vi "REC_ThermalCAM.vi"() -> ()   [LabVIEW 2018]
doc: "To use this browser, you can type in a URL in the location field and then click on the Go button. You can also use the Back, Forward, Reload and Search buttons. This VI also has a runtime menu which is included in the library. When you run the VI, you will have File Menu and a History Menu. The file menu contains the same functionality that the buttons can do and the History menu contains a History of all the pages that you have visited in a given session.\n\nThe Invoke Node and Property Node functions are used to control the operation of the web browser. For more information on the Microsoft Web Browser Control, see Microsoft's web site (try http://support.microsoft.com/support/kb/articles/q165/2/12.asp)."
panel:
  out "Passing Array":string[](array[string])=["http://espn.go.com/", "http://www.natinst.com/"]
  in  "Search":bool
  in  "Go":bool
  in  "Reload":bool
  in  "Back":bool
  in  "Forward":bool
  in  "URL :":string="192.168.1.65"
  in  "SHDocVw.IWebBrowser2":refnum<k7>(container)
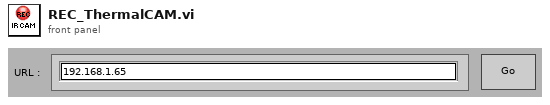
[diagram p1: front panel]
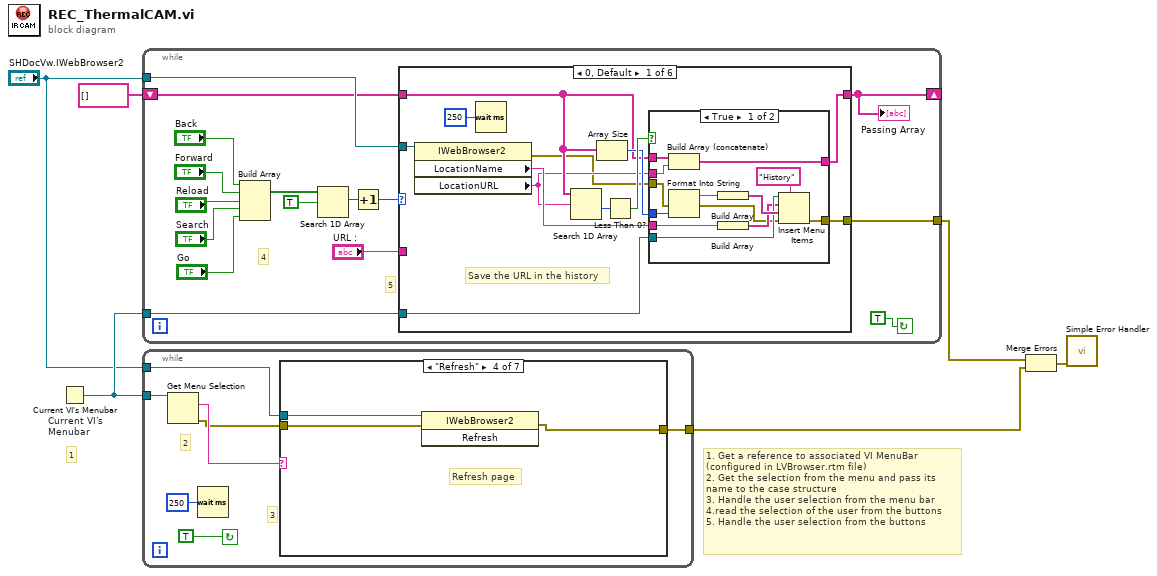
[diagram p0: block diagram]
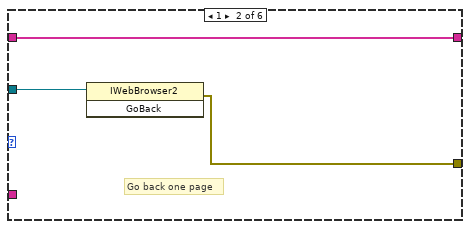
[diagram p3: hidden frame]
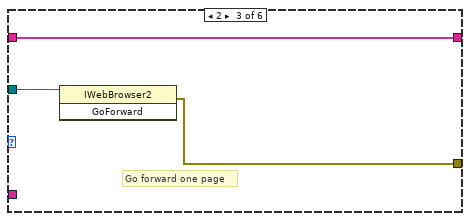
[diagram p4: hidden frame]
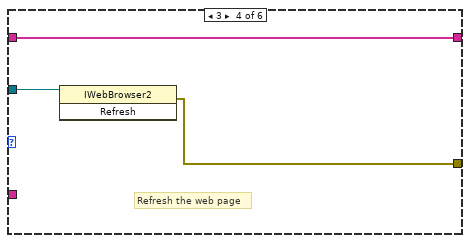
[diagram p5: hidden frame]
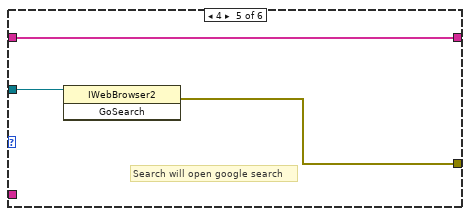
[diagram p6: hidden frame]
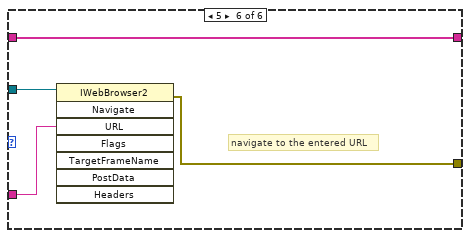
[diagram p7: hidden frame]
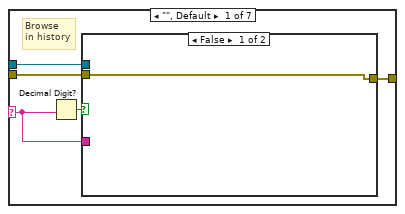
[diagram p8: hidden frame]
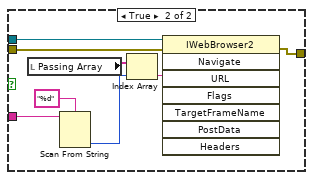
[diagram p9: hidden frame]
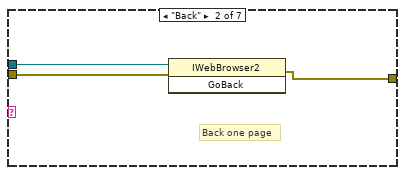
[diagram p10: hidden frame]
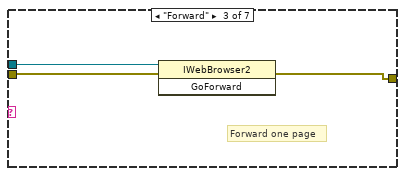
[diagram p11: hidden frame]
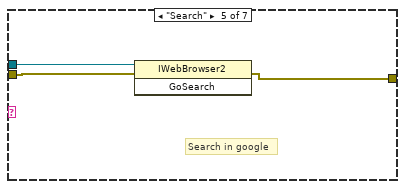
[diagram p12: hidden frame]
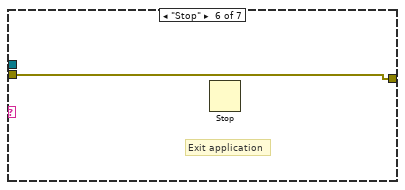
[diagram p13: hidden frame]
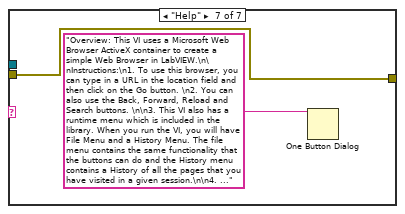
[diagram p14: hidden frame]
diagram:
  # "1. Get a reference to associated VI MenuBar \n(configured in LVBrowser.rtm file)\n2. Get the selection from the menu and pass its \nname to the case structure\n3. Handle the user selection from the menu bar\n4.read the selection of the user from the buttons\n5. Handle the user selection from the buttons"
  # "1"
  n1 = Current VI's Menubar "Current VI's \nMenubar"() -> (w6:refnum<k9>)
  n2 = while {
    shift-left: string[] [] -> [w9]
    shift-right: [w8] -> _
    tunnel: w6 -> [w10]
    tunnel: "SHDocVw.IWebBrowser2" -> [w12]
    tunnel: [w7] -> w3
    stop <- TRUE continue-if-true
    # "5"
    # "4"
    n3 = Build Array("Back", "Forward", "Reload", "Search", "Go") -> (w16:bool[])
    n4 = Search 1D Array(1D array=w16, element=TRUE) -> (index of element=w14:i32)  [unwired: 1 in]
    n5 = Increment(x=w14) -> (x+1=w13:i32)
    n6 = case shown="0, Default" w13 {
      tunnel: w12 -> [w25 w52 w55 w57 w60 w65]
      tunnel: "URL :" -> [_ _ _ _ _ w64]
      tunnel: w10 -> [w26 _ _ _ _ _]
      tunnel: w9 -> [w30 w51 w54 w58 w61 w63]
      tunnel: [w29 w51 w54 w58 w61 w63] -> w8
      tunnel: [w24 w50 w53 w56 w59 w62] -> w7
      frame 0, Default {
        # "Save the URL in the history"
        n7 = property class="IWebBrowser2"(reference=w25) -> (error out=w23:errorcluster, "LocationName"=w34:string, "LocationURL"=w27:string)  [unwired: 1 in, 1 out]
        n8 = Wait (ms)(milliseconds to wait=u32 250 ("millisecond multiple")) -> ()  [unwired: 1 out]
        n9 = Search 1D Array(1D array=w30, element=w27) -> (index of element=w33:i32)  [unwired: 1 in]
        n10 = Array Size(array=w30) -> (size(s)=w31:i32)
        n11 = Less Than 0?(x=w33) -> (x < 0?=w32:bool)
        n12 = case shown="True" w32 {
          tunnel: w26 -> [w44 _]
          tunnel: w34 -> [w42 _]
          tunnel: w27 -> [w38 _]
          tunnel: w31 -> [w39 _]
          tunnel: w30 -> [w41 w49]
          tunnel: [w40 w49] -> w29
          tunnel: [w36 w48] -> w24
          tunnel: w23 -> [w35 w48]
          frame True {
            n13 = Build Array (concatenate)(w41, w38) -> (w40:string[])
            n14 = Format Into String(error in=w35, w39) -> (resulting string=w47:string, error out=w37:errorcluster)  [unwired: 2 in]
            n15 = Build Array(w47) -> (w46:string[])
            n16 = Build Array(w42) -> (w43:string[])
            n17 = Insert Menu Items(5:"History" ("menu tag"), 6:w37, 7:w46, 8:w43, 9:w44) -> (0:w36:errorcluster)  [unwired: 1 in, 2 out]
          }
          frame False {
          }
        }
      }
      frame 1 {
        # "Go back one page"
        n18 = invoke class="IWebBrowser2" method="GoBack"(reference=w52) -> (error out=w50:errorcluster)  [unwired: 2 in, 2 out]
      }
      frame 2 {
        # "Go forward one page"
        n19 = invoke class="IWebBrowser2" method="GoForward"(reference=w55) -> (error out=w53:errorcluster)  [unwired: 2 in, 2 out]
      }
      frame 3 {
        # "Refresh the web page"
        n20 = invoke class="IWebBrowser2" method="Refresh"(reference=w57) -> (error out=w56:errorcluster)  [unwired: 2 in, 2 out]
      }
      frame 4 {
        # "Search will open google search"
        n21 = invoke class="IWebBrowser2" method="GoSearch"(reference=w60) -> (error out=w59:errorcluster)  [unwired: 2 in, 2 out]
      }
      frame 5 {
        # "navigate to the entered URL"
        n22 = invoke class="IWebBrowser2" method="Navigate"(reference=w65, "URL"=w64) -> (error out=w62:errorcluster)  [unwired: 6 in, 7 out]
      }
    }
    "Passing Array" <- w8
  }
  n23 = while {
    tunnel: w6 -> [w71]
    tunnel: "SHDocVw.IWebBrowser2" -> [w69]
    tunnel: [w66] -> w2
    stop <- TRUE continue-if-true
    # "3"
    # "2"
    n24 = Get Menu Selection(0:w71) -> (6:w70:string, 8:w67:errorcluster)  [unwired: 3 in, 3 out]
    n25 = Wait (ms)(milliseconds to wait=u32 250 ("millisecond multiple")) -> ()  [unwired: 1 out]
    n26 = case shown="\"Refresh\"" w70 {
      selector: w70 -> [w75 _ _ _ _ _ _]
      tunnel: w69 -> [w77 w89 w92 w95 w98 _ _]
      tunnel: w67 -> [w74 w88 w91 w94 w97 w99 w100]
      tunnel: [w73 w87 w90 w93 w96 w99 w100] -> w66
      frame "", Default {
        # "Browse\nin history"
        n27 = Decimal Digit?(1:w75) -> (0:w76:bool)
        n28 = case shown="False" w76 {
          tunnel: w77 -> [_ w86]
          tunnel: w75 -> [_ w82]
          tunnel: w74 -> [w78 w80]
          tunnel: [w78 w79] -> w73
          frame False {
          }
          frame True {
            n29 = local read "Passing Array"() -> (w85:string[])
            n30 = Scan From String(format string="%d", input string=w82) -> (output 1=w81:i32)  [unwired: 3 in, 3 out]
            n31 = Index Array(array=w85, index=w81) -> (element=w84:string)
            n32 = invoke class="IWebBrowser2" method="Navigate"(reference=w86, error in=w80, "URL"=w84) -> (error out=w79:errorcluster)  [unwired: 5 in, 7 out]
          }
        }
      }
      frame "Back" {
        # "Back one page"
        n33 = invoke class="IWebBrowser2" method="GoBack"(reference=w89, error in=w88) -> (error out=w87:errorcluster)  [unwired: 1 in, 2 out]
      }
      frame "Forward" {
        # "Forward one page"
        n34 = invoke class="IWebBrowser2" method="GoForward"(reference=w92, error in=w91) -> (error out=w90:errorcluster)  [unwired: 1 in, 2 out]
      }
      frame "Refresh" {
        # "Refresh page"
        n35 = invoke class="IWebBrowser2" method="Refresh"(reference=w95, error in=w94) -> (error out=w93:errorcluster)  [unwired: 1 in, 2 out]
      }
      frame "Search" {
        # "Search in google"
        n36 = invoke class="IWebBrowser2" method="GoSearch"(reference=w98, error in=w97) -> (error out=w96:errorcluster)  [unwired: 1 in, 2 out]
      }
      frame "Stop" {
        # "Exit application"
        n37 = Stop() -> ()  [unwired: 1 in]
      }
      frame "Help" {
        n38 = One Button Dialog(message="Overview: This VI uses a Microsoft Web Browser ActiveX container to create a simple Web Browser in LabVIEW.\n\nInstructions:\n1. To use this browser, you can type in a URL in the location field and then click on the Go button. \n2. You can also use the Back, Forward, Reload and Search buttons. \n\n3. This VI also has a runtime menu which is included in the library. When you run the VI, you will have File Menu and a History Menu. The file menu contains the same functionality that the buttons can do and the History menu contains a History of all the pages that you have visited in a given session.\n\n4. To Stop Execution, Click on File>> Stop") -> ()  [unwired: 1 in, 1 out]
      }
    }
  }
  n39 = Merge Errors(w3, w2) -> (w1:errorcluster)
  n40 = call <vilib>:"Simple Error Handler.vi"("error in (no error)"=w1) -> ()  [unwired: 4 in, 5 out]
